vi "Tile naming.vi"(7 "?":T1=enum."Increment slice", 8 "Error In":errorcluster) -> (0 "Error Out":errorcluster, 2 "tile":i32, 3 "slice":i32)   [LabVIEW 2018]
uses:
  Controls/Tile naming actions.ctl
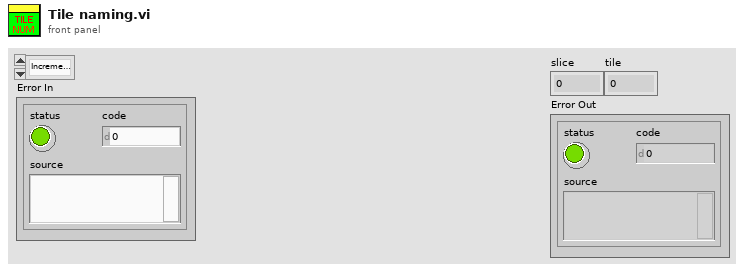
[diagram p1: front panel]
types:
  T1 = typedef "Tile naming actions.ctl" = enum16{"Export", "Increment slice", "Increment tile", "Init"}
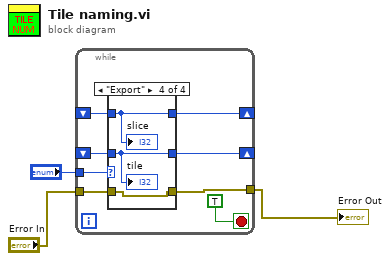
[diagram p0: block diagram]
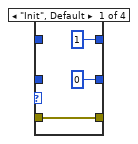
[diagram p2: hidden frame]
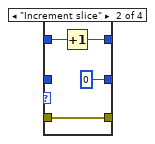
[diagram p3: hidden frame]
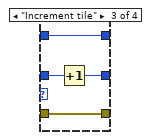
[diagram p4: hidden frame]
diagram:
  n1 = while {
    tunnel: "?" -> [w11]
    shift-right: [w9] -> _
    shift-left: _ -> [w7]
    shift-right: [w10] -> _
    shift-left: _ -> [w6]
    tunnel: "Error In" -> [w5]
    tunnel: [w4] -> w1
    stop <- TRUE stop-if-true
    n2 = case shown="\"Export\"" w11 {
      tunnel: [0 0 w21 w24] -> w10
      tunnel: [1 w17 w20 w25] -> w9
      tunnel: w7 -> [_ w18 w20 w25]
      tunnel: w6 -> [_ _ w22 w24]
      tunnel: w5 -> [w12 w15 w19 w23]
      tunnel: [w12 w15 w19 w23] -> w4
      frame "Init", Default {
      }
      frame "Increment slice" {
        n3 = Increment(x=w18) -> (x+1=w17:i32)
      }
      frame "Increment tile" {
        n4 = Increment(x=w22) -> (x+1=w21:i32)
      }
      frame "Export" {
        "slice" <- w25
        "tile" <- w24
      }
    }
  }
  "Error Out" <- w1
